vi "Global.vi"() -> ()   [LabVIEW 2018]
panel:
  out "Decals Ref":refnum<vi>
  in  "Abort":bool
  in  "Current Step":u8
  in  "# of Steps":u8
  # "PROGRESS BAR INPUTS"
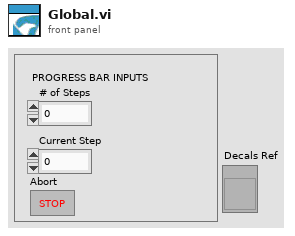
[diagram p1: front panel]
diagram:
